vi "DialogAddDesignPattern.vi"(0 "ClassWriter in":refnum<class "ClassWriter.lvclass">, 1 "ClassItemRefIn":refnum<vi>, 5 "error in (no error)":errorcluster) -> (14 "ClassWriter out":refnum<class "ClassWriter.lvclass">, 15 "ClassItemRefOut":refnum<vi>, 16 "CreateMethodData":T1, 17 "Cancelled":bool, 19 "error out":errorcluster)   [LabVIEW 2020, in "ClassWriter.lvclass"]
uses:
  <resource>/Framework/Providers/Open_GDS/ClassProviders/Provider_BaseClassInterface/ClassWriter_class/ClassWriter.lvclass
  <resource>/Framework/Providers/Open_GDS/ClassProviders/Provider_BaseClassInterface/AddDesignPatternData.ctl
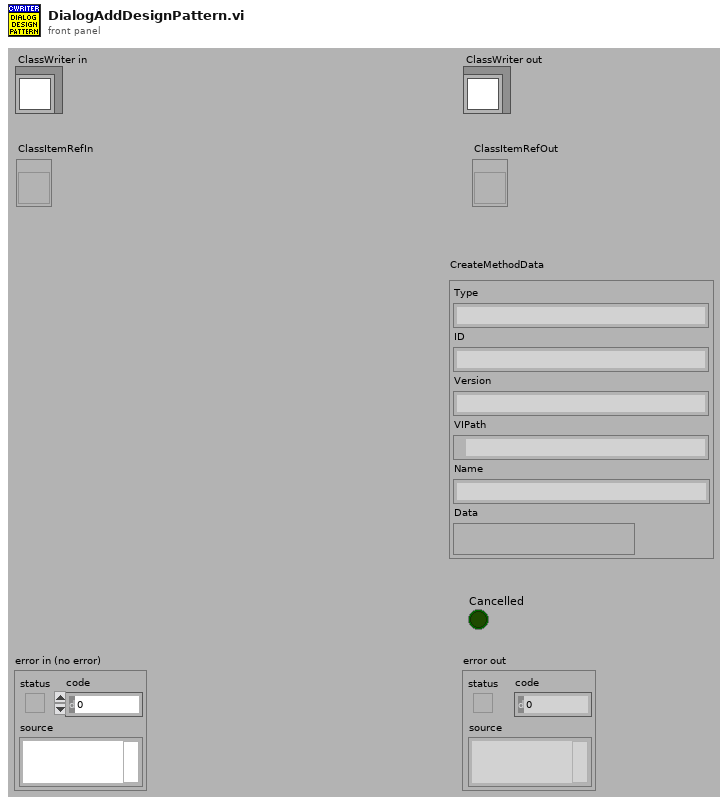
[diagram p1: front panel]
types:
  T1 = typedef "AddDesignPatternData.ctl" = cluster{"Type":string, "ID":string, "Version":string, "VIPath":path, "Name":string, "Data":variant}
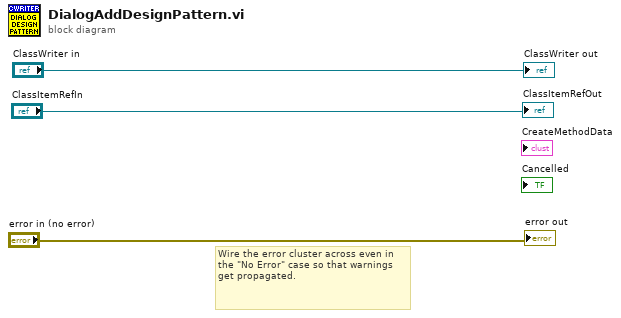
[diagram p0: block diagram]
diagram:
  # "Wire the error cluster across even in the \"No Error\" case so that warnings get propagated."
  "error out" <- "error in (no error)"
  "ClassWriter out" <- "ClassWriter in"
  "ClassItemRefOut" <- "ClassItemRefIn"
